vi "Table.vi"(4 "Result Cell Configuration":T7={"Cell Defaults"={"Background Color"=16777215, "Horizontal Align"=3, "Vertical Align"=1, "Minimum Height"=0.0, "Fixed Height"=0.0, "Padding"={"Left"=2.0, "Top"=2.0, "Right"=2.0, "Bottom"=3.0}}, "Borders"={"Left"={"Enabled"=TRUE, "Width"=0.5, "Color"=0}, "Top"={"Enabled"=TRUE, "Width"=0.75, "Color"=0}, "Right"={"Enabled"=TRUE, "Width"=1.0, "Color"=0}, "Bottom"={"Enabled"=TRUE, "Width"=0.75, "Color"=0}}, "Column Span"=0} {"Cell Defaults"."Vertical Align" items=["Bottom", "Middle", "Top"]; "Cell Defaults"."Horizontal Align" items=["Center", "Justified", "JustifiedAll", "Left", "Right"]}, 5 "Row Configuration":T10={"Cell Defaults"={"Background Color"=16777215, "Horizontal Align"=3, "Vertical Align"=1, "Minimum Height"=0.0, "Fixed Height"=0.0, "Padding"={"Left"=2.0, "Top"=2.0, "Right"=2.0, "Bottom"=3.0}}, "Row Borders"={"Left"={"Enabled"=TRUE, "Width"=0.5, "Color"=0}, "Top"={"Enabled"=TRUE, "Width"=0.75, "Color"=0}, "Right"={"Enabled"=TRUE, "Width"=0.5, "Color"=0}, "Bottom"={"Enabled"=TRUE, "Width"=0.75, "Color"=0}, "Middle Vertical"={"Enabled"=TRUE, "Width"=0.5, "Color"=0}}} {"Cell Defaults"."Vertical Align" items=["Bottom", "Middle", "Top"]; "Cell Defaults"."Horizontal Align" items=["Center", "Justified", "JustifiedAll", "Left", "Right"]}, 6 "Font":T13={"Font"="Arial", "Size"=10, "Colour"=0, "Bold"=FALSE, "Italic"=FALSE, "Underline"=FALSE, "Strikethrough"=FALSE, "Font Encoding"=enum."Cp1252, WinANSI"}, 7 "Table Configuration":T11={"Table Settings"={"Number of Columns"=6, "Width (%)"=100.0, "Relative Column Widths (%)"=[10.0, 30.0, 20.0, 15.0, 15.0, 10.0], "Horizontal Align"=0, "Header Rows"=1}, "Cell Defaults"={"Background Color"=16777215, "Horizontal Align"=3, "Vertical Align"=1, "Minimum Height"=0.0, "Fixed Height"=0.0, "Padding"={"Left"=2.0, "Top"=2.0, "Right"=2.0, "Bottom"=3.0}}, "Borders"={"Left"={"Enabled"=TRUE, "Width"=1.0, "Color"=0}, "Top"={"Enabled"=TRUE, "Width"=1.0, "Color"=0}, "Right"={"Enabled"=TRUE, "Width"=1.0, "Color"=0}, "Bottom"={"Enabled"=TRUE, "Width"=1.0, "Color"=0}, "Middle Horizontal"={"Enabled"=TRUE, "Width"=0.5, "Color"=0}, "Middle Vertical"={"Enabled"=TRUE, "Width"=0.5, "Color"=0}}} {"Cell Defaults"."Vertical Align" items=["Bottom", "Middle", "Top"]; "Cell Defaults"."Horizontal Align" items=["Center", "Justified", "JustifiedAll", "Left", "Right"]; "Table Settings"."Horizontal Align" items=["Center"=0, "Left"=3, "Right"=4]}, 8 "error in":errorcluster, 10 "Table Content":T1={"TableHeader"=["Soll\nppm/%", "Ist\nppm/%", "Fehler\n%", "Toleranz\n%", "Ergebnis"], "Table"=[], "Relative Column Widths (%)"=[], "Results"={"Results"=[], "ResultPictures"={"Yes Ctl Refnum"=refnum, "No Ctl Refnum"=refnum}, "use Pictures"=FALSE, "Image Scale (%)"=100.0, "Autoscale? (T)"=TRUE, "Horizontal Align"=3, "Position"=0}, "PositionBemerkung"=enum."before", "PageBreak"=enum."before", "TablePictures"={"Ctl Refnum In"=[], "RowOrColumn"=enum."Row", "IndexToInsert"=0, "Image Scale (%)"=[], "Autoscale? (T)"=[], "Horizontal Align"=3}, "Horizontal Align"=3} {"Horizontal Align" items=["Center", "Justified", "JustifiedAll", "Left", "Right"]; "TablePictures"."Horizontal Align" items=["Center", "Justified", "JustifiedAll", "Left", "Right"]; "Results"."Position" items=["First", "Last"]; "Results"."Horizontal Align" items=["Center", "Justified", "JustifiedAll", "Left", "Right"]}, 11 "Context In":refnum<class "Context.lvclass">=refnum) -> (0 "error out":errorcluster, 3 "Context Out":refnum<class "Context.lvclass">)   [LabVIEW 2020, in "PDF Interface.lvlib" / "PDF Interface Helper.lvlib"]
uses:
  PDF Interface Helper.lvlib
  <vilib>/Simplicity AI/SAI_PDF_API/Classes/Context/Controls/SAI_PDF_Font.ctl
  <vilib>/Simplicity AI/SAI_PDF_API/Classes/Context/Controls/SAI_PDF_Font Encoding.ctl
  <vilib>/Simplicity AI/SAI_PDF_API/Classes/Context/Context.lvclass
  <vilib>/Simplicity AI/SAI_PDF_API/Classes/Table Builder/Controls/SAI_PDF_Table Configuration.ctl
  <vilib>/Simplicity AI/SAI_PDF_API/Classes/Table Builder/Controls/SAI_PDF_Table Horizontal Align.ctl
  <vilib>/Simplicity AI/SAI_PDF_API/Classes/Table Builder/Controls/SAI_PDF_Default Cell Format.ctl
  <vilib>/Simplicity AI/SAI_PDF_API/Classes/Table Builder/Controls/SAI_PDF_BorderLine.ctl
  <vilib>/Simplicity AI/SAI_PDF_API/Classes/Table Builder/Controls/SAI_PDF_Row Configuration.ctl
  <vilib>/Simplicity AI/SAI_PDF_API/Classes/Table Builder/Controls/SAI_PDF_Cell Configuration.ctl
  PDFTableContentType.ctl
  PDFResults.ctl
  PDFResultPictures.ctl
  PDFCommentPosition.ctl
  PDFPageBreak.ctl
  PDFTablePictures.ctl
  <vilib>/Simplicity AI/SAI_PDF_API/Classes/Table Builder/Table Builder.lvclass
panel:
  # "(Cp1252)"
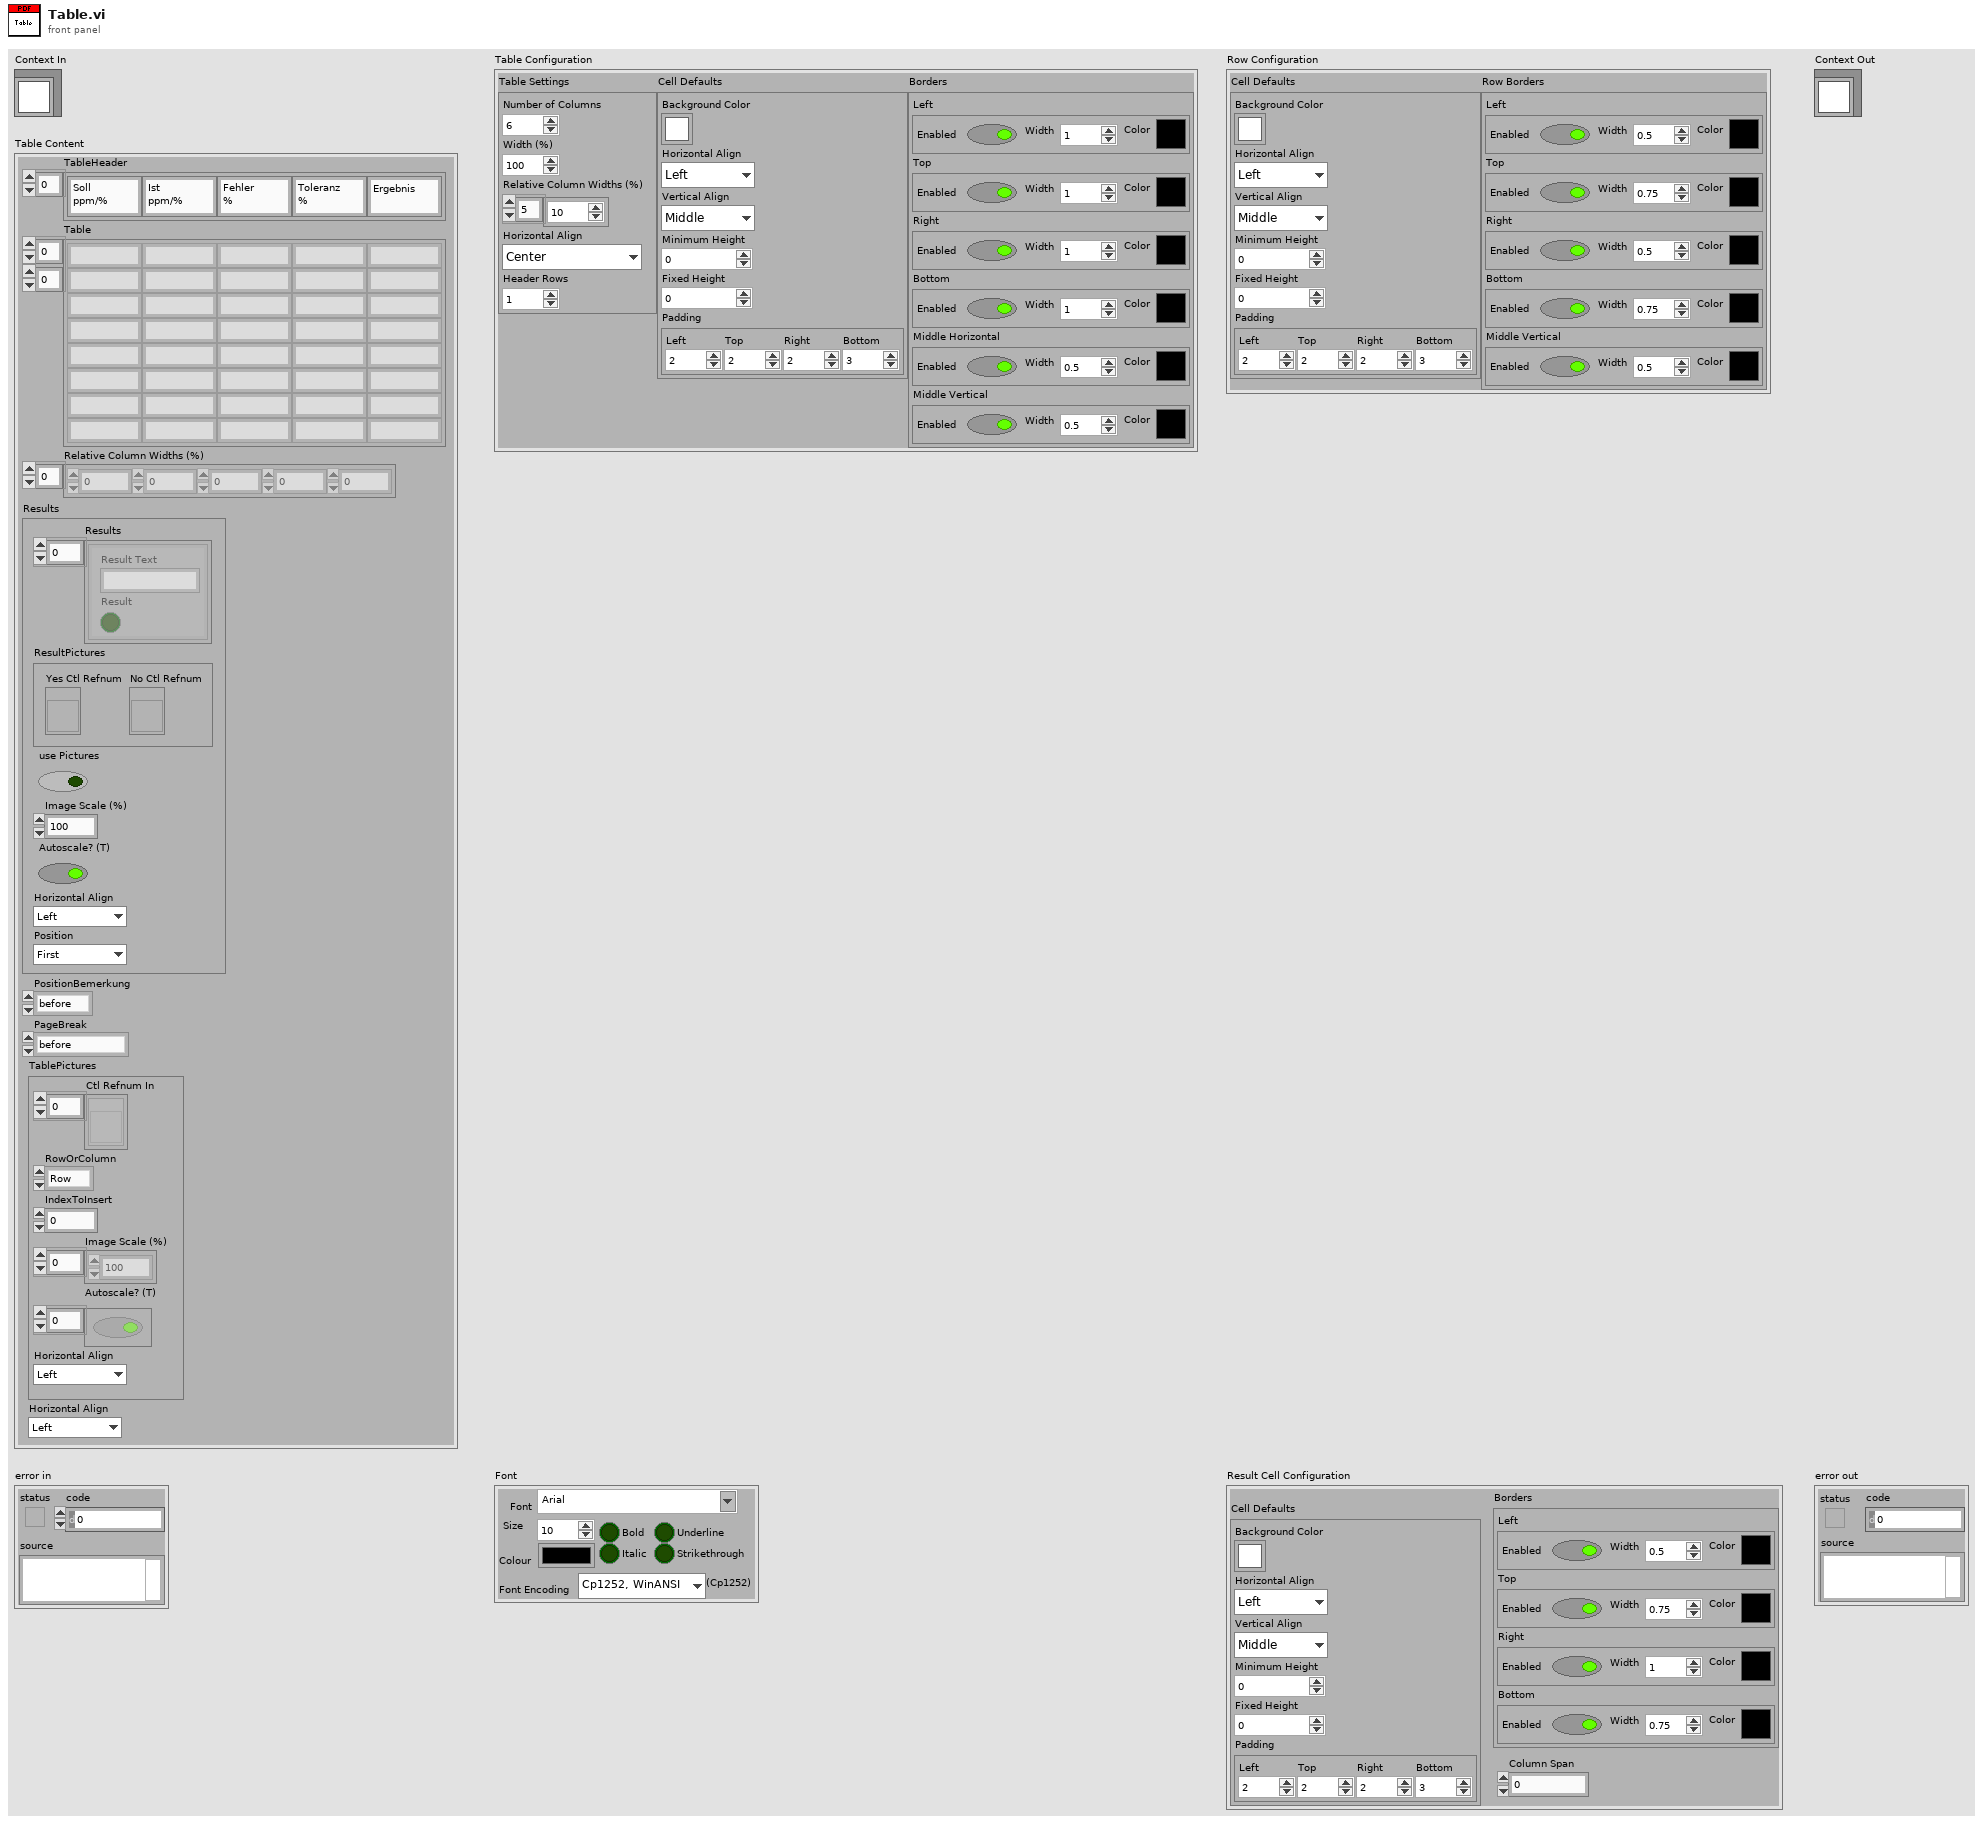
[diagram p1: front panel]
types:
  T1 = typedef "PDF Interface.lvlib/PDF Interface Helper.lvlib/PDFTableContentType.ctl" = cluster{"TableHeader":string[], "Table":string[][], "Relative Column Widths (%)":sgl[], "Results":T2, "PositionBemerkung":T4, "PageBreak":T5, "TablePictures":T6, "Horizontal Align":i32}
  T2 = typedef "PDF Interface.lvlib/PDF Interface Helper.lvlib/PDFResults.ctl" = cluster{"Results":cluster{"Result Text":string, "Result":bool}[], "ResultPictures":T3, "use Pictures":bool, "Image Scale (%)":sgl, "Autoscale? (T)":bool, "Horizontal Align":i32, "Position":i32}
  T3 = typedef "PDF Interface.lvlib/PDF Interface Helper.lvlib/PDFResultPictures.ctl" = cluster{"Yes Ctl Refnum":refnum<vi>, "No Ctl Refnum":refnum<vi>}
  T4 = typedef "PDF Interface.lvlib/PDF Interface Helper.lvlib/PDFCommentPosition.ctl" = enum16{"before", "after"}
  T5 = typedef "PDF Interface.lvlib/PDF Interface Helper.lvlib/PDFPageBreak.ctl" = enum16{"none", "before", "after", "after comment"}
  T6 = typedef "PDF Interface.lvlib/PDF Interface Helper.lvlib/PDFTablePictures.ctl" = cluster{"Ctl Refnum In":refnum<vi>[], "RowOrColumn":enum16{"Row", "Column"}, "IndexToInsert":u16, "Image Scale (%)":sgl[], "Autoscale? (T)":bool[], "Horizontal Align":i32}
  T7 = typedef "SAI_PDF_Toolkit.lvlib/Table Builder.lvclass/SAI_PDF_Cell Configuration.ctl" = cluster{"Cell Defaults":T8, "Borders":cluster{"Left":T9, "Top":T9, "Right":T9, "Bottom":T9}, "Column Span":i32}
  T8 = typedef "SAI_PDF_Toolkit.lvlib/Table Builder.lvclass/SAI_PDF_Default Cell Format.ctl" = cluster{"Background Color":u32, "Horizontal Align":i32, "Vertical Align":i32, "Minimum Height":sgl, "Fixed Height":sgl, "Padding":cluster{"Left":sgl, "Top":sgl, "Right":sgl, "Bottom":sgl}}
  T9 = typedef "SAI_PDF_Toolkit.lvlib/Table Builder.lvclass/SAI_PDF_BorderLine.ctl" = cluster{"Enabled":bool, "Width":sgl, "Color":u32}
  T10 = typedef "SAI_PDF_Toolkit.lvlib/Table Builder.lvclass/SAI_PDF_Row Configuration.ctl" = cluster{"Cell Defaults":T8, "Row Borders":cluster{"Left":T9, "Top":T9, "Right":T9, "Bottom":T9, "Middle Vertical":T9}}
  T11 = typedef "SAI_PDF_Toolkit.lvlib/Table Builder.lvclass/SAI_PDF_Table Configuration.ctl" = cluster{"Table Settings":cluster{"Number of Columns":i32, "Width (%)":sgl, "Relative Column Widths (%)":sgl[], "Horizontal Align":T12, "Header Rows":i32}, "Cell Defaults":T8, "Borders":cluster{"Left":T9, "Top":T9, "Right":T9, "Bottom":T9, "Middle Horizontal":T9, "Middle Vertical":T9}}
  T12 = typedef "SAI_PDF_Toolkit.lvlib/Table Builder.lvclass/SAI_PDF_Table Horizontal Align.ctl" = i32
  T13 = typedef "SAI_PDF_Toolkit.lvlib/Context.lvclass/SAI_PDF_Font.ctl" = cluster{"Font":string, "Size":i32, "Colour":u32, "Bold":bool, "Italic":bool, "Underline":bool, "Strikethrough":bool, "Font Encoding":T14}
  T14 = typedef "SAI_PDF_Toolkit.lvlib/Context.lvclass/SAI_PDF_Font Encoding.ctl" = enum16{"Cp1252, WinANSI", "IdentityH", "IdentityV", "Cp1250", "Cp1257", "MacRoman"}
  T15 = cluster{"TablePictures empty?":bool, "TableHeader empty?":bool, "Results empty?":bool, "Table empty?":bool}
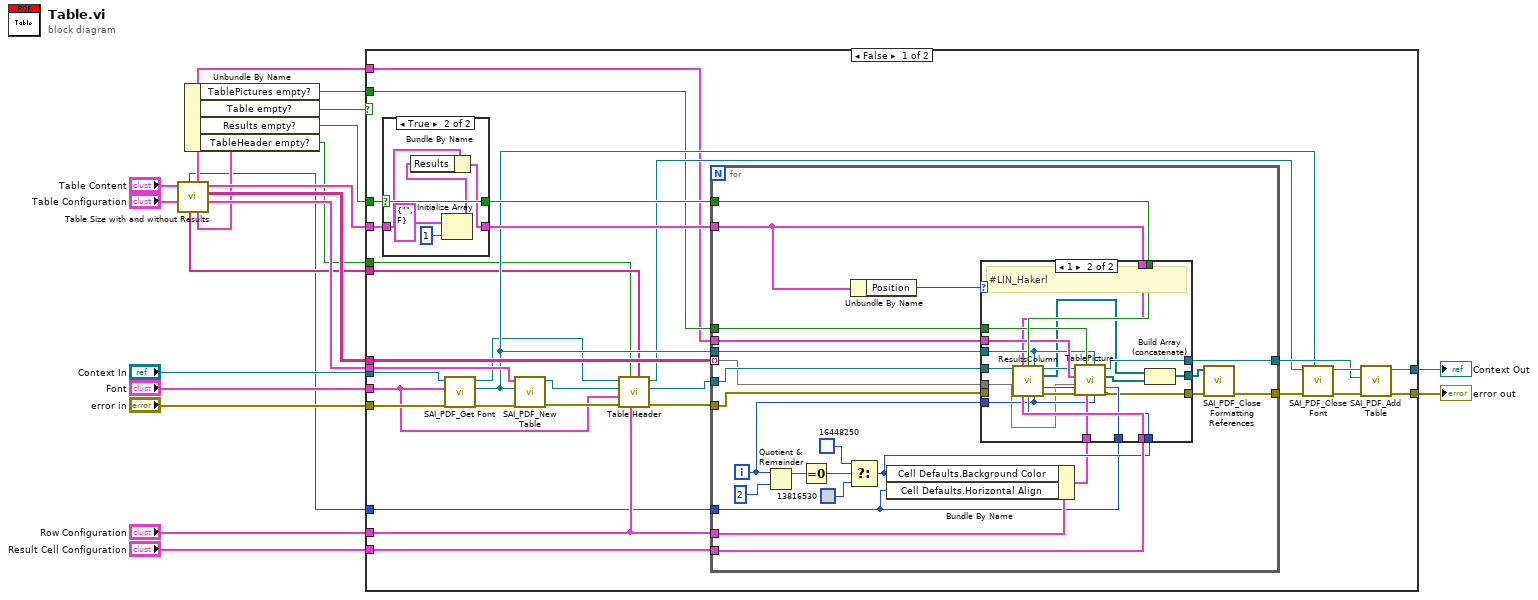
[diagram p0: block diagram]
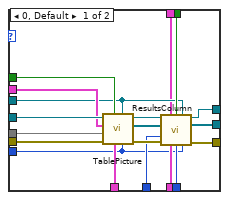
[diagram p3: hidden frame]
diagram:
  n1 = call "Table Size with and without Results.vi"("Table Configuration (Eingang)"="Table Configuration", "Table Content"="Table Content") -> ("Table Configuration (Ausgang)"=w14:T11, "Table out"=w13:string[][], "Results out"=w12:T2, "Empty-Cluster"=w6:T15, "TablePictures out"=w2:T6, "TableHeader out"=w10:string[], "Horizontal Align"=w1:i32)  [unwired: 2 in, 1 out]
  n2 = Unbundle By Name(w6) -> ("TablePictures empty?"=w3:bool, "Table empty?"=w7:bool, "Results empty?"=w5:bool, "TableHeader empty?"=w4:bool)
  n3 = case shown="False" w7 {
    tunnel: "error in" -> [w50 w121]
    tunnel: "Context In" -> [w49 w122]
    tunnel: [w45 w122] -> w18
    tunnel: [w44 w121] -> w17
    tunnel: "Result Cell Configuration" -> [w43 _]
    tunnel: w14 -> [w38 _]
    tunnel: w13 -> [w37 _]
    tunnel: w5 -> [w36 _]
    tunnel: w12 -> [w35 _]
    tunnel: w10 -> [w33 _]
    tunnel: w4 -> [w27 _]
    tunnel: "Font" -> [w25 _]
    tunnel: "Row Configuration" -> [w24 _]
    tunnel: w3 -> [w23 _]
    tunnel: w2 -> [w22 _]
    tunnel: w1 -> [w21 _]
    frame False {
      n4 = case shown="True" w36 {
        selector: w36 -> [w52 w56]
        tunnel: [w51 w53] -> w40
        tunnel: [w52 w56] -> w39
        tunnel: w35 -> [w51 w55]
        frame False {
        }
        frame True {
          n5 = Initialize Array(cluster{"Result Text":string, "Result":bool} {"Result Text"="", "Result"=FALSE} ("Results"), 1 ("Dimensionsgröße")) -> (w54:cluster{"Result Text":string, "Result":bool}[])
          n6 = Bundle By Name(cluster=w55, "Results"=w54) -> (w53:T2)
        }
      }
      n7 = call <vilib>:"SAI_PDF_Get Font.vi"("error in"=w50, "Font"=w25, "Context In"=w49) -> ("error out"=w48:errorcluster, "Font"=w34:refnum<class "Font.lvclass">, "Context Out"=w32:refnum<class "Context.lvclass">)  [unwired: 6 out]
      n8 = call <vilib>:"SAI_PDF_New Table.vi"("error in"=w48, "Font In"=w34, "Table Configuration"=w38) -> ("error out"=w31:errorcluster, "Table Builder"=w26:refnum<class "Table Builder.lvclass">)  [unwired: 7 out]
      n9 = call "Table Header.vi"("TableHeader out"=w33, "Row Configuration"=w24, "TableHeader empty?"=w27, "Fehler (Eingang, kein Fehler)"=w31, "Font"=w25, "Table Builder (Eingang)"=w26, "Context (Eingang)"=w32) -> ("Fehler (Ausgang)"=w29:errorcluster, "Table Builder (Ausgang)"=w30:refnum<class "Table Builder.lvclass">, "Context (Ausgang)"=w28:refnum<class "Context.lvclass">)  [unwired: 2 in]
      n10 = for {
        tunnel: w30 -> [w82]
        tunnel: w29 -> [w79]
        tunnel: [w80] -> w41
        tunnel: w37 -> [w81] mode=indexing
        tunnel: w40 -> [w60]
        tunnel: w34 -> [w62]
        tunnel: w24 -> [w73]
        tunnel: w43 -> [w72]
        tunnel: [w70] -> w42
        tunnel: w39 -> [w69]
        tunnel: w23 -> [w66]
        tunnel: w22 -> [w67]
        tunnel: w21 -> [w64]
        i -> [w61]
        n11 = Quotient & Remainder(x=w61, y=2) -> (x-y*floor(x/y)=w77:i32)  [unwired: 1 out]
        n12 = Equal To 0?(x=w77) -> (x = 0?=w76:bool)
        n13 = Select(t=u32 16448250, s=w76, f=u32 13816530) -> (s? t:f=w68:u32)
        n14 = Unbundle By Name(w60) -> ("Position"=w59:i32)
        n15 = Bundle By Name(cluster=w73, "Cell Defaults.Background Color"=w68, "Cell Defaults.Horizontal Align"=w64) -> (w65:T10)
        n16 = case shown="1" w59 {
          tunnel: w82 -> [w101 w110]
          tunnel: w81 -> [w100 w105]
          tunnel: [w99 w108] -> w80
          tunnel: w79 -> [w97 _]
          tunnel: w72 -> [w96 w120]
          tunnel: [w95 w106] -> w71
          tunnel: w69 -> [w94 w119]
          tunnel: w68 -> [w93 w118]
          tunnel: w67 -> [w92 w117]
          tunnel: w66 -> [w91 w116]
          tunnel: w65 -> [w90 w115]
          tunnel: w64 -> [w88 w114]
          tunnel: [w87 w103] -> w63
          tunnel: w62 -> [w86 w113]
          tunnel: w61 -> [w84 w112]
          tunnel: w60 -> [w83 w111]
          frame 0, Default {
            n17 = call "TablePicture.vi"("RowIndex"=w84, "Font In"=w86, "Row Configuration"=w90, "TablePictures empty?"=w91, "Fehler (Eingang, kein Fehler)"=w97, "Table in"=w100, "TablePictures in"=w92, "Table Builder (Eingang)"=w101) -> ("Fehler (Ausgang)"=w98:errorcluster, "Row Formatting out"=w89:refnum<class "Formatting.lvclass">[], "Table Builder (Ausgang)"=w85:refnum<class "Table Builder.lvclass">)  [unwired: 1 in]
            n18 = call "ResultsColumn.vi"("Table Builder (Eingang)"=w85, "Results out"=w83, "empty?"=w94, "Font (Eingang)"=w86, "Row Formatting in"=w89, "Horizontal Align"=w88, "Fehler (Eingang, kein Fehler)"=w98, "Result Cell Configuration"=w96, "BackgroundColor"=w93, "RowIndex"=w84) -> ("Table Builder (Ausgang)"=w99:refnum<class "Table Builder.lvclass">, "Row Formatting Array out"=w87:refnum<class "Formatting.lvclass">[], "Fehler (Ausgang)"=w95:errorcluster)  [unwired: 3 in]
          }
          frame 1 {
            # "#LIN_Hakerl"
            n19 = call "ResultsColumn.vi"("Table Builder (Eingang)"=w110, "Results out"=w111, "empty?"=w119, "Font (Eingang)"=w113, "Horizontal Align"=w114, "Result Cell Configuration"=w120, "BackgroundColor"=w118, "RowIndex"=w112) -> ("Table Builder (Ausgang)"=w109:refnum<class "Table Builder.lvclass">, "Row Formatting Array out"=w102:refnum<class "Formatting.lvclass">[], "Fehler (Ausgang)"=w107:errorcluster)  [unwired: 5 in]
            n20 = call "TablePicture.vi"("RowIndex"=w112, "Font In"=w113, "Row Configuration"=w115, "TablePictures empty?"=w116, "Fehler (Eingang, kein Fehler)"=w107, "Table in"=w105, "TablePictures in"=w117, "Table Builder (Eingang)"=w109) -> ("Fehler (Ausgang)"=w106:errorcluster, "Row Formatting out"=w104:refnum<class "Formatting.lvclass">[], "Table Builder (Ausgang)"=w108:refnum<class "Table Builder.lvclass">)  [unwired: 1 in]
            n21 = Build Array (concatenate)(w102, w104) -> (w103:refnum<class "Formatting.lvclass">[])
          }
        }
        n22 = call <vilib>:"SAI_PDF_Close Formatting References.vi"("error in"=w71, "Formatting Refs"=w63) -> ("error out"=w70:errorcluster)  [unwired: 9 out]
      }
      n23 = call <vilib>:"SAI_PDF_Close Font.vi"("Font"=w34, "error in"=w42, "Context In"=w28) -> ("error out"=w46:errorcluster, "Context Out"=w47:refnum<class "Context.lvclass">)  [unwired: 7 out]
      n24 = call <vilib>:"SAI_PDF_Add Table.vi"("error in"=w46, "Table Builder In"=w41, "Context In"=w47) -> ("error out"=w44:errorcluster, "Context Out"=w45:refnum<class "Context.lvclass">)  [unwired: 7 out]
    }
    frame True {
    }
  }
  "error out" <- w17
  "Context Out" <- w18
